vi "OPCConnection.Properties.vi"(7 "Action":enum8{"Get", "Set"}(ring), 8 "error in (no error)":errorcluster, 10 "Connection.Properties":T1={"Server IP Address"="localhost", "Server Port"=49350, "Message Mode"=enum."None", "Security"=enum."Basic256", "User Name"="", "Password"="", "Client Certificate"=path "", "Server Certificate"=path "", "Server Certificate (RT)"=path "", "Client Certificate (RT)"=path ""}, 11 "Item Ref in":T2 format="%.0x") -> (0 "error out":errorcluster, 2 "Connection.Properties":T1={"Server IP Address"="localhost", "Server Port"=49350, "Message Mode"=enum."None", "Security"=enum."Basic256", "User Name"="", "Password"="", "Client Certificate"=path "", "Server Certificate"=path "", "Server Certificate (RT)"=path "", "Client Certificate (RT)"=path ""}, 3 "Item Ref out":T2 format="%.0x")   [LabVIEW 2019, in "OPC UA Client Addon System Explorer.lvlib"]
uses:
  OPC UA Client Addon System Explorer.lvlib
  <vilib>/NI VeriStand/Custom Device API/Custom Device Item Ref.ctl
  Addon Shared/Types/OPCConnection.Properties.ctl
  <vilib>/NI VeriStand/Custom Device API/Dependent File Optional Info.ctl
  Addon Shared/SubVIs/Constants.vi
  <vilib>/NI VeriStand/Custom Device API/Get Item Property (String).vi
  <vilib>/NI VeriStand/Custom Device API/Get Item Property (U16).vi
  <vilib>/NI VeriStand/Custom Device API/Get Item Property (Dependent File).vi
  <vilib>/NI VeriStand/Custom Device API/Set Item Property (String).vi
  <vilib>/NI VeriStand/Custom Device API/Set Item Property (U16).vi
  <vilib>/NI VeriStand/Custom Device API/Set Item Property (Dependent File).vi
  <vilib>/NI VeriStand/Custom Device API/Custom Device API.lvlib
  Addon Shared/OPC UA Client Addon Shared.lvlib
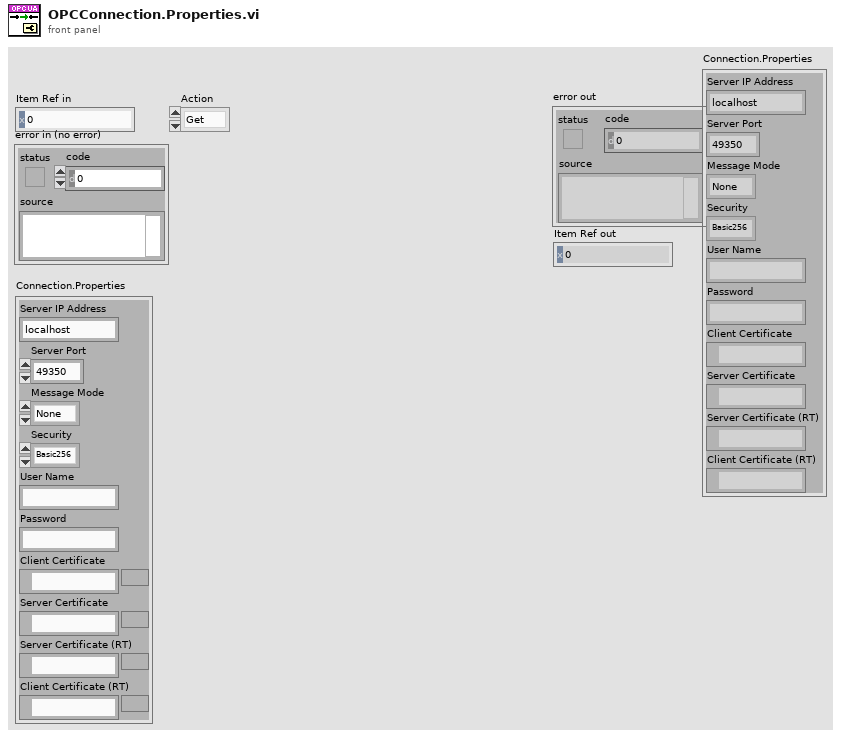
[diagram p1: front panel]
types:
  T1 = typedef "OPC UA Client Addon Shared.lvlib/OPCConnection.Properties.ctl" = cluster{"Server IP Address":string, "Server Port":u16, "Message Mode":enum16{"None", "Sign", "Sign and Encrypt"}, "Security":enum16{"Basic256", "Basic128Rsa15"}, "User Name":string, "Password":string, "Client Certificate":path, "Server Certificate":path, "Server Certificate (RT)":path, "Client Certificate (RT)":path}
  T2 = typedef "Custom Device API.lvlib/Custom Device Item Ref.ctl" = u64
  T3 = typedef "Custom Device API.lvlib/Dependent File Optional Info.ctl" = cluster{"Version":string, "RTDestination":path, "ForceDownload":bool, "SupportedTarget":string, "MD5":string}
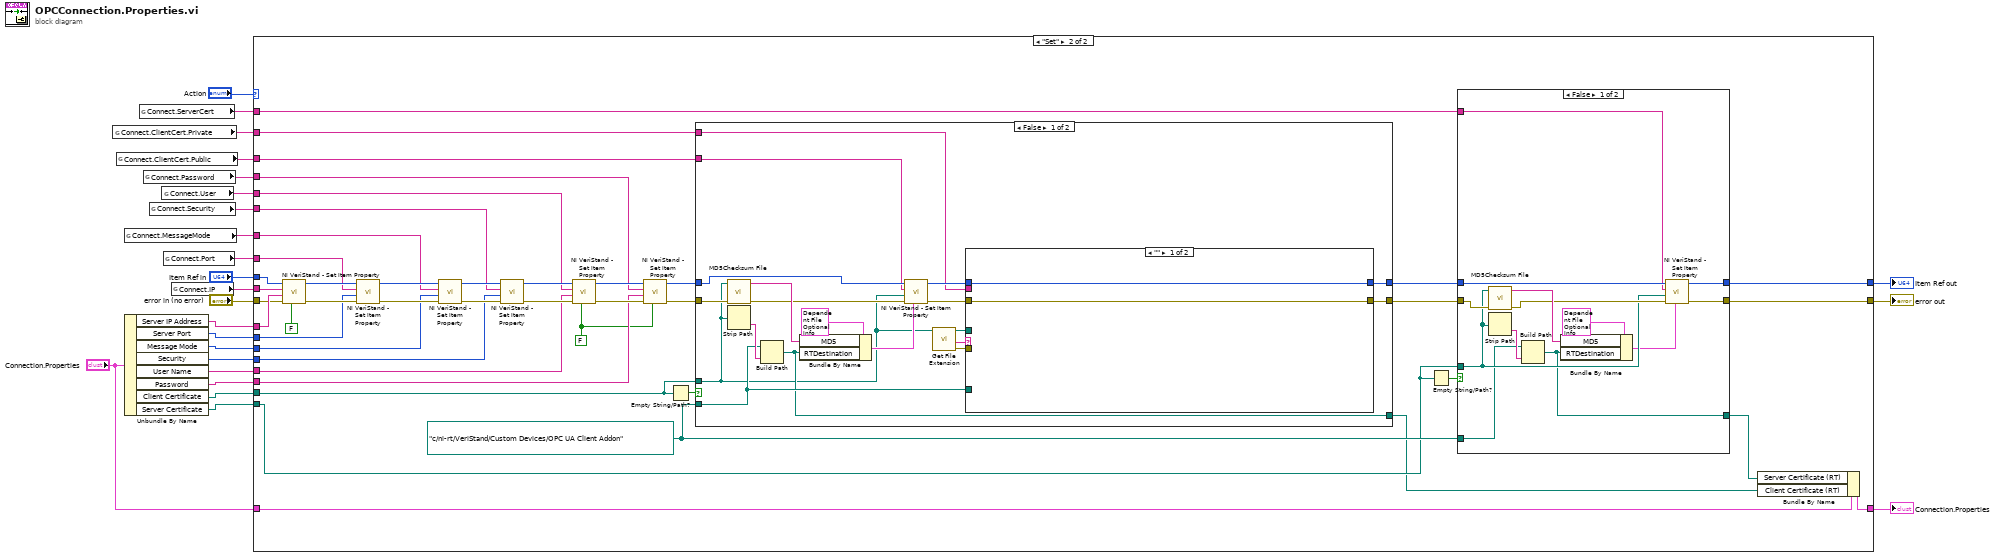
[diagram p0: block diagram]
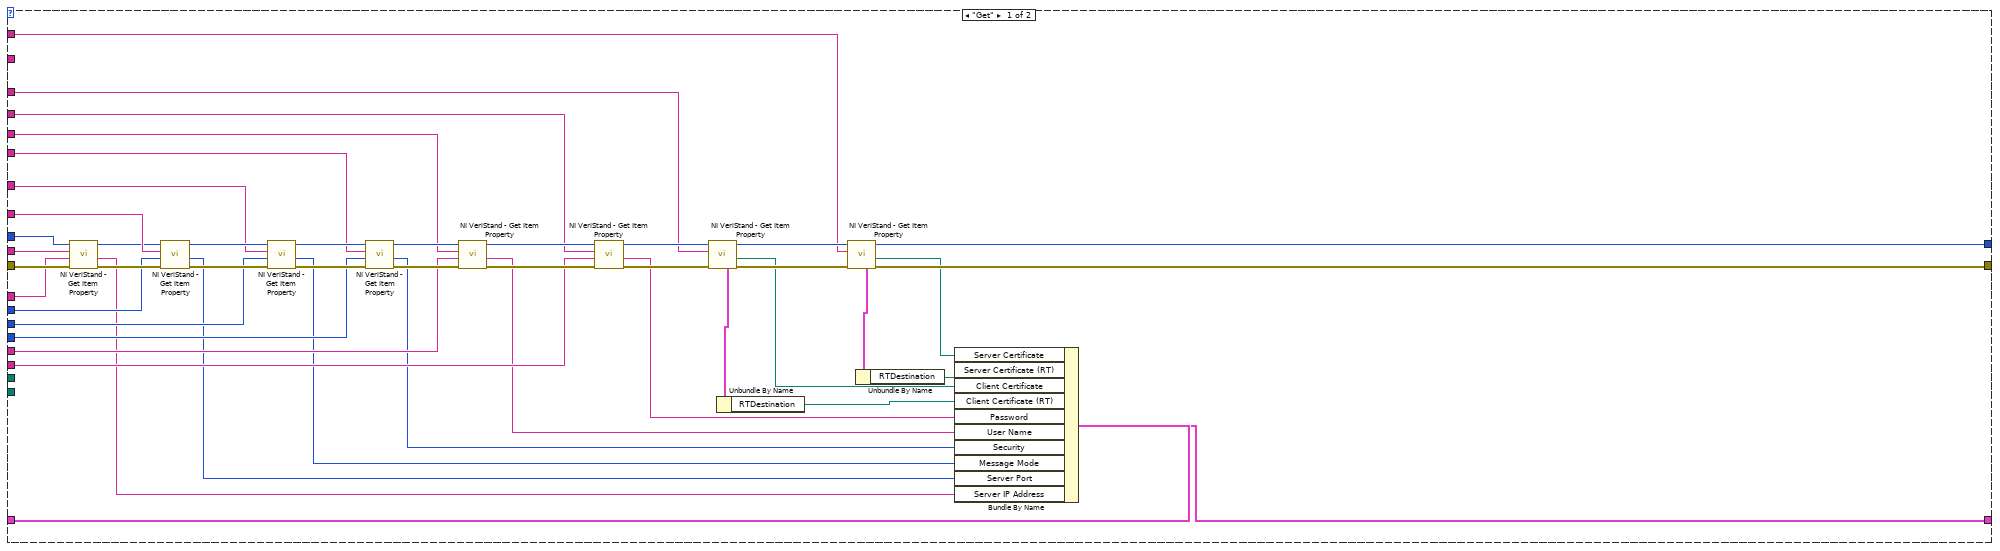
[diagram p2: hidden frame]
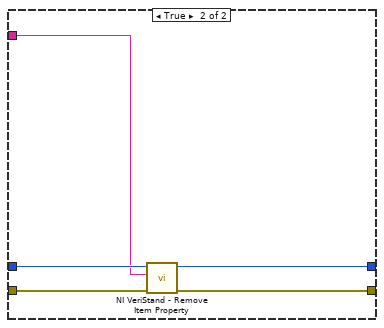
[diagram p3: hidden frame]
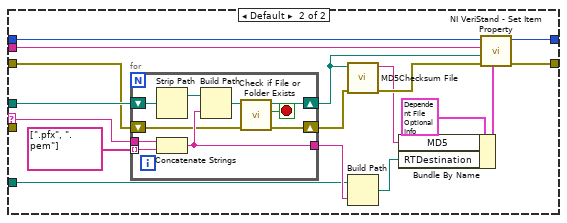
[diagram p4: hidden frame]
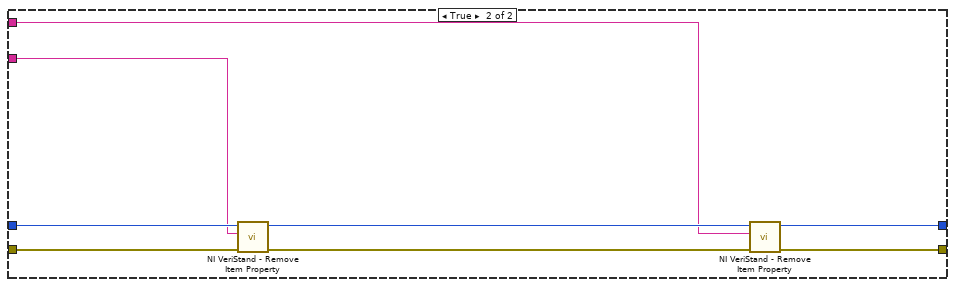
[diagram p5: hidden frame]
diagram:
  n1 = global read "Constants.vi" "Connect.ClientCert.Private"() -> (w15:string)
  n2 = global read "Constants.vi" "Connect.ClientCert.Public"() -> (w14:string)
  n3 = global read "Constants.vi" "Connect.MessageMode"() -> (w12:string)
  n4 = Unbundle By Name("Connection.Properties") -> ("Server IP Address"=w23:string, "Server Port"=w22:u16, "Message Mode"=w21:enum16{"None", "Sign", "Sign and Encrypt"}, "Security"=w20:enum16{"Basic256", "Basic128Rsa15"}, "User Name"=w19:string, "Password"=w18:string, "Client Certificate"=w4:path, "Server Certificate"=w17:path)
  n5 = global read "Constants.vi" "Connect.ServerCert"() -> (w16:string)
  n6 = global read "Constants.vi" "Connect.Password"() -> (w10:string)
  n7 = global read "Constants.vi" "Connect.Security"() -> (w13:string)
  n8 = global read "Constants.vi" "Connect.User"() -> (w11:string)
  n9 = global read "Constants.vi" "Connect.Port"() -> (w5:string)
  n10 = global read "Constants.vi" "Connect.IP"() -> (w24:string)
  n11 = case shown="\"Set\"" "Action" {
    tunnel: w24 -> [w61 w114]
    tunnel: w23 -> [w52 w101]
    tunnel: w22 -> [w51 w100]
    tunnel: w21 -> [w50 w99]
    tunnel: w20 -> [w49 w98]
    tunnel: w19 -> [w48 w97]
    tunnel: w18 -> [w47 w96]
    tunnel: w17 -> [_ w75]
    tunnel: w16 -> [w39 w80]
    tunnel: w15 -> [_ w95]
    tunnel: w14 -> [w40 w94]
    tunnel: w13 -> [w43 w93]
    tunnel: w12 -> [w44 w92]
    tunnel: w11 -> [w42 w91]
    tunnel: w10 -> [w41 w90]
    tunnel: [w46 w78] -> w9
    tunnel: [w45 w79] -> w8
    tunnel: "Item Ref in" -> [w62 w87]
    tunnel: "error in (no error)" -> [w70 w86]
    tunnel: w5 -> [w60 w85]
    tunnel: w4 -> [_ w84]
    tunnel: "Connection.Properties" -> [w38 w74]
    tunnel: [w29 w71] -> w2
    frame "Get" {
      n12 = call-poly <vilib>:"NI VeriStand - Get Item Property.vi"("error in (no error)"=w70, "Default Value"=w52, "Property Name"=w61, "Item Ref in"=w62) -> ("error out"=w69:errorcluster, "Value"=w33:string, "Item Ref out"=w59:T2)  [unwired: 4 in, 1 out]
      n13 = call-poly <vilib>:"NI VeriStand - Get Item Property.vi"("error in (no error)"=w69, "Default Value"=w51, "Property Name"=w60, "Item Ref in"=w59) -> ("error out"=w68:errorcluster, "Value"=w32:u16, "Item Ref out"=w58:T2)  [unwired: 4 in, 1 out]
      n14 = call-poly <vilib>:"NI VeriStand - Get Item Property.vi"("error in (no error)"=w68, "Default Value"=w50, "Property Name"=w44, "Item Ref in"=w58) -> ("error out"=w67:errorcluster, "Value"=w31:u16, "Item Ref out"=w57:T2)  [unwired: 4 in, 1 out]
      n15 = call-poly <vilib>:"NI VeriStand - Get Item Property.vi"("error in (no error)"=w67, "Default Value"=w49, "Property Name"=w43, "Item Ref in"=w57) -> ("error out"=w66:errorcluster, "Value"=w30:u16, "Item Ref out"=w56:T2)  [unwired: 4 in, 1 out]
      n16 = call-poly <vilib>:"NI VeriStand - Get Item Property.vi"("error in (no error)"=w66, "Default Value"=w48, "Property Name"=w42, "Item Ref in"=w56) -> ("error out"=w65:errorcluster, "Value"=w34:string, "Item Ref out"=w55:T2)  [unwired: 4 in, 1 out]
      n17 = call-poly <vilib>:"NI VeriStand - Get Item Property.vi"("error in (no error)"=w65, "Default Value"=w47, "Property Name"=w41, "Item Ref in"=w55) -> ("error out"=w64:errorcluster, "Value"=w35:string, "Item Ref out"=w54:T2)  [unwired: 4 in, 1 out]
      n18 = call-poly <vilib>:"NI VeriStand - Get Item Property.vi"("error in (no error)"=w64, "Property Name"=w40, "Item Ref in"=w54) -> ("error out"=w63:errorcluster, "Path"=w36:path, "Item Ref out"=w53:T2, "OptionalInfo"=w28:T3)  [unwired: 4 in, 1 out]
      n19 = Unbundle By Name(w28) -> ("RTDestination"=w27:path)
      n20 = call-poly <vilib>:"NI VeriStand - Get Item Property.vi"("error in (no error)"=w63, "Property Name"=w39, "Item Ref in"=w53) -> ("error out"=w46:errorcluster, "Path"=w37:path, "Item Ref out"=w45:T2, "OptionalInfo"=w26:T3)  [unwired: 4 in, 1 out]
      n21 = Unbundle By Name(w26) -> ("RTDestination"=w25:path)
      n22 = Bundle By Name(cluster=w38, "Server Certificate"=w37, "Server Certificate (RT)"=w25, "Client Certificate"=w36, "Client Certificate (RT)"=w27, "Password"=w35, "User Name"=w34, "Security"=w30, "Message Mode"=w31, "Server Port"=w32, "Server IP Address"=w33) -> (w29:T1)
    }
    frame "Set" {
      w77 = path "c:/ni-rt/VeriStand/Custom Devices/OPC UA Client Addon" ("RTDestination")
      w89 = FALSE ("Binary String (T)")
      n23 = call-poly <vilib>:"NI VeriStand - Set Item Property.vi"("Binary String (T)"=FALSE, "error in (no error)"=w86, "Value"=w101, "Property Name"=w114, "Item Ref in"=w87) -> ("error out"=w107:errorcluster, "Item Ref out"=w113:T2)  [unwired: 4 in, 1 out]
      n24 = call-poly <vilib>:"NI VeriStand - Set Item Property.vi"("error in (no error)"=w107, "Value"=w100, "Property Name"=w85, "Item Ref in"=w113) -> ("error out"=w106:errorcluster, "Item Ref out"=w112:T2)  [unwired: 5 in, 1 out]
      n25 = call-poly <vilib>:"NI VeriStand - Set Item Property.vi"("error in (no error)"=w106, "Value"=w99, "Property Name"=w92, "Item Ref in"=w112) -> ("error out"=w105:errorcluster, "Item Ref out"=w111:T2)  [unwired: 5 in, 1 out]
      n26 = call-poly <vilib>:"NI VeriStand - Set Item Property.vi"("error in (no error)"=w105, "Value"=w98, "Property Name"=w93, "Item Ref in"=w111) -> ("error out"=w104:errorcluster, "Item Ref out"=w110:T2)  [unwired: 5 in, 1 out]
      n27 = call-poly <vilib>:"NI VeriStand - Set Item Property.vi"("Binary String (T)"=w89, "error in (no error)"=w104, "Value"=w97, "Property Name"=w91, "Item Ref in"=w110) -> ("error out"=w103:errorcluster, "Item Ref out"=w109:T2)  [unwired: 4 in, 1 out]
      n28 = call-poly <vilib>:"NI VeriStand - Set Item Property.vi"("Binary String (T)"=w89, "error in (no error)"=w103, "Value"=w96, "Property Name"=w90, "Item Ref in"=w109) -> ("error out"=w102:errorcluster, "Item Ref out"=w108:T2)  [unwired: 4 in, 1 out]
      n29 = Empty String/Path?(string/path=w84) -> (empty?=w83:bool)
      n30 = case shown="False" w83 {
        tunnel: w108 -> [w151 w184]
        tunnel: w102 -> [w139 w187]
        tunnel: [w149 w183] -> w81
        tunnel: w95 -> [w148 w181]
        tunnel: w94 -> [w147 w182]
        tunnel: [w145 w186] -> w82
        tunnel: w84 -> [w133 _]
        tunnel: w77 -> [w136 _]
        tunnel: [w135 _] -> w72
        frame False {
          n31 = call <vilib>:"MD5Checksum File.vi"("error in (no error)"=w139, "Path"=w133) -> ("error out"=w138:errorcluster, "MD5 message-digest"=w140:string)  [unwired: 8 in]
          n32 = Strip Path(path=w133) -> (name=w142:string)  [unwired: 1 out]
          n33 = Build Path(base path=w136, name or relative path=w142) -> (appended path=w135:path)
          n34 = Bundle By Name(cluster=T3 {"Version"="1.0", "RTDestination"=path "c:/ni-rt/VeriStand/Custom Devices/FPGA Addon", "ForceDownload"=FALSE, "SupportedTarget"="All", "MD5"=""} ("OptionalInfo"), "MD5"=w140, "RTDestination"=w135) -> (w137:T3)
          n35 = call-poly <vilib>:"NI VeriStand - Set Item Property.vi"("OptionalInfo"=w137, "error in (no error)"=w138, "Path"=w133, "Property Name"=w147, "Item Ref in"=w151) -> ("error out"=w146:errorcluster, "Item Ref out"=w150:T2)  [unwired: 4 in, 1 out]
          n36 = call <vilib>:"Get File Extension.vi"("file"=w133) -> ("error out"=w143:errorcluster, "filename without extension"=w144:string, "dup file"=w134:path)  [unwired: 6 in, 2 out]
          n37 = case shown="\"\"" w144 {
            selector: w144 -> [_ w166]
            tunnel: w150 -> [w152 w170]
            tunnel: [w152 w169] -> w149
            tunnel: w148 -> [_ w168]
            tunnel: w146 -> [w153 w155]
            tunnel: [w153 w167] -> w145
            tunnel: w143 -> [_ _]
            tunnel: w134 -> [_ w158]
            tunnel: w136 -> [_ w160]
            frame "" {
            }
            frame Default {
              n38 = for {
                tunnel: w166 -> [w180]
                shift-right: [w174] -> w157
                shift-left: w158 -> [w177]
                shift-right: [w173] -> w156
                shift-left: w155 -> [w172]
                tunnel: string[] [".pfx", ".pem"] -> [w179] mode=indexing
                tunnel: [w178] -> w161
                stop <- w171 stop-if-true
                n39 = Strip Path(path=w177) -> (stripped path=w176:path)  [unwired: 1 out]
                n40 = Concatenate Strings(w180, w179) -> (w178:string)
                n41 = Build Path(base path=w176, name or relative path=w178) -> (appended path=w175:path)
                n42 = call <vilib>:"Check if File or Folder Exists.vi"("error in (no error)"=w172, "path"=w175) -> ("error out"=w173:errorcluster, "file or folder exists?"=w171:bool, "dup path"=w174:path)  [unwired: 7 in]
              }
              n43 = call <vilib>:"MD5Checksum File.vi"("error in (no error)"=w156, "Path"=w157) -> ("error out"=w165:errorcluster, "MD5 message-digest"=w163:string)  [unwired: 8 in]
              n44 = Build Path(base path=w160, name or relative path=w161) -> (appended path=w159:path)
              n45 = Bundle By Name(cluster=T3 {"Version"="1.0", "RTDestination"=path "c:/ni-rt/VeriStand/Custom Devices/FPGA Addon", "ForceDownload"=FALSE, "SupportedTarget"="All", "MD5"=""} ("OptionalInfo"), "MD5"=w163, "RTDestination"=w159) -> (w162:T3)
              n46 = call-poly <vilib>:"NI VeriStand - Set Item Property.vi"("OptionalInfo"=w162, "error in (no error)"=w165, "Path"=w157, "Property Name"=w168, "Item Ref in"=w170) -> ("error out"=w167:errorcluster, "Item Ref out"=w169:T2)  [unwired: 4 in, 1 out]
            }
          }
        }
        frame True {
          n47 = call <vilib>:"NI VeriStand - Remove Item Property.vi"("error in (no error)"=w187, "Property Name"=w182, "Item Ref in"=w184) -> ("error out"=w188:errorcluster, "Item Ref out"=w185:T2)  [unwired: 6 in, 1 out]
          n48 = call <vilib>:"NI VeriStand - Remove Item Property.vi"("error in (no error)"=w188, "Property Name"=w181, "Item Ref in"=w185) -> ("error out"=w186:errorcluster, "Item Ref out"=w183:T2)  [unwired: 6 in, 1 out]
        }
      }
      n49 = Empty String/Path?(string/path=w75) -> (empty?=w76:bool)
      n50 = case shown="False" w76 {
        tunnel: w81 -> [w127 w130]
        tunnel: w82 -> [w122 w132]
        tunnel: w80 -> [w126 w128]
        tunnel: w75 -> [w120 _]
        tunnel: w77 -> [w118 _]
        tunnel: [w117 w129] -> w79
        tunnel: [w116 w131] -> w78
        tunnel: [w115 _] -> w73
        frame False {
          n51 = call <vilib>:"MD5Checksum File.vi"("error in (no error)"=w122, "Path"=w120) -> ("error out"=w121:errorcluster, "MD5 message-digest"=w123:string)  [unwired: 8 in]
          n52 = Strip Path(path=w120) -> (name=w125:string)  [unwired: 1 out]
          n53 = Build Path(base path=w118, name or relative path=w125) -> (appended path=w115:path)
          n54 = Bundle By Name(cluster=T3 {"Version"="1.0", "RTDestination"=path "c:/ni-rt/VeriStand/Custom Devices/FPGA Addon", "ForceDownload"=FALSE, "SupportedTarget"="All", "MD5"=""} ("OptionalInfo"), "MD5"=w123, "RTDestination"=w115) -> (w119:T3)
          n55 = call-poly <vilib>:"NI VeriStand - Set Item Property.vi"("OptionalInfo"=w119, "error in (no error)"=w121, "Path"=w120, "Property Name"=w126, "Item Ref in"=w127) -> ("error out"=w116:errorcluster, "Item Ref out"=w117:T2)  [unwired: 4 in, 1 out]
        }
        frame True {
          n56 = call <vilib>:"NI VeriStand - Remove Item Property.vi"("error in (no error)"=w132, "Property Name"=w128, "Item Ref in"=w130) -> ("error out"=w131:errorcluster, "Item Ref out"=w129:T2)  [unwired: 6 in, 1 out]
        }
      }
      n57 = Bundle By Name(cluster=w74, "Server Certificate (RT)"=w73, "Client Certificate (RT)"=w72) -> (w71:T1)
    }
  }
  "error out" <- w9
  "Item Ref out" <- w8
  "Connection.Properties" <- w2
